vi "Create Channel.vi"(6 "index":i32, 8 "error in":errorcluster, 10 "channel settings":T1, 11 "analog input mode in":refnum<class "Analog Input Mode.lvclass">) -> (0 "error out":errorcluster, 2 "analog input channel":refnum<class "AI Channel.lvclass">, 3 "analog input mode out":refnum<class "Analog Input Mode.lvclass">)   [LabVIEW 2017, in "Scan Engine Scripting.lvlib" / "Analog Input Mode.lvclass"]
uses:
  Analog Input Mode.lvclass
  Controls/analog channel settings.ctl
  Channel Classes/AI Channel/AI Channel.lvclass
  Analog Input Mode.lvclass/Analog Input Mode.ctl
  Scan Engine Scripting.lvlib
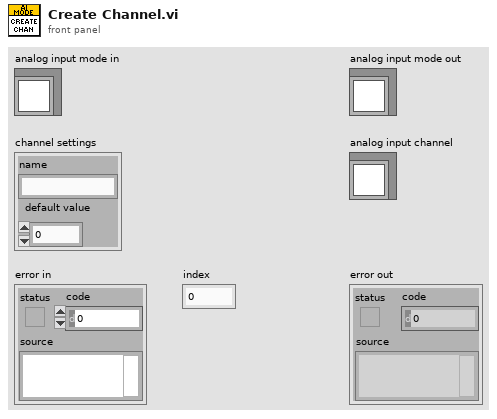
[diagram p1: front panel]
types:
  T1 = typedef "Scan Engine Scripting.lvlib/analog channel settings.ctl" = cluster{"name":string, "default value":dbl}
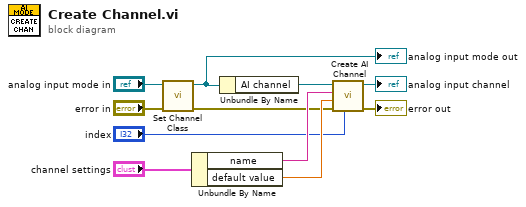
[diagram p0: block diagram]
diagram:
  n1 = call-dynamic "Set Channel Class.vi"("error in"="error in", "analog input mode in"="analog input mode in") -> ("error out"=w2:errorcluster, "analog input mode out"=w1:refnum<class "Analog Input Mode.lvclass">)  [unwired: 8 in]
  "analog input mode out" <- w1
  n2 = Unbundle By Name("channel settings") -> ("name"=w9:string, "default value"=w8:dbl)
  n3 = Unbundle By Name(w1) -> ("AI channel"=w10:refnum<class "AI Channel.lvclass">)
  n4 = call-dynamic "Create AI Channel.vi"("index"="index", "error in"=w2, "default value"=w8, "name"=w9, "AI channel in"=w10) -> ("error out"=→"error out":errorcluster, "AI channel out"=→"analog input channel":refnum<class "AI Channel.lvclass">)  [unwired: 5 in]
